vi "AlliGator Is SS2 Dataset HDF5 File.vi"(7 "File Path":path, 9 "Error In":errorcluster) -> (8 "Is SS2 Dataset?":bool, 10 "Error Out":errorcluster)   [LabVIEW 2021, in "AlliGator HDF5.lvlib"]
doc: "Checks wether a HDF5 file is a SS2 dataset file (early version)."
uses:
  AlliGator HDF5.lvlib
  <vilib>/addons/h5labview2/base/lib_path.vi
  <vilib>/addons/h5labview2/base/H5Equery.vi
  <vilib>/addons/h5labview2/base/hid_t.ctl
  <vilib>/addons/h5labview2/dataset/H5Dread.llb/H5Dread.xnode
  <vilib>/addons/h5labview2/file/H5F.lvlib
panel:
  # "see the AlliGator License on the block diagram (Ctrl+E or Window:Show Block Diagram)"
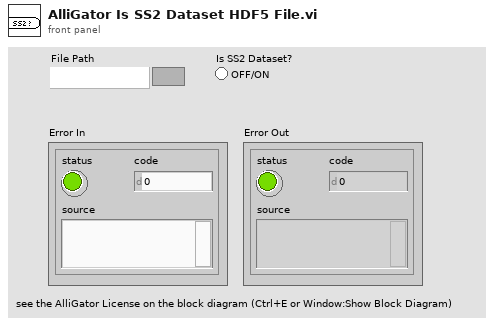
[diagram p1: front panel]
types:
  T1 = typedef "hid_t.ctl" = i64
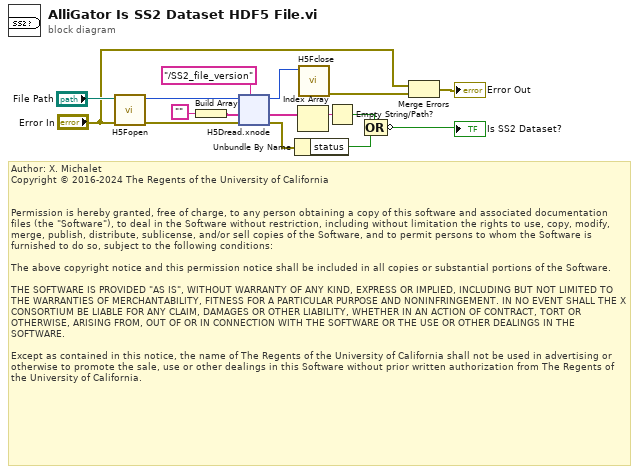
[diagram p0: block diagram]
diagram:
  # "Author: X. Michalet\nCopyright © 2016-2024 The Regents of the University of California\n \n\nPermission is hereby granted, free of charge, to any person obtaining a copy of this software and associated documentation files (the \"Software\"), to deal in the Software without restriction, including without limitation the rights to use, copy, modify, merge, publish, distribute, sublicense, and/or sell copies of the Software, and to permit persons to whom the Software is furnished to do so, subject to the following conditions:\n\nThe above copyright notice and this permission notice shall be included in all copies or substantial portions of the Software.\n\nTHE SOFTWARE IS PROVIDED \"AS IS\", WITHOUT WARRANTY OF ANY KIND, EXPRESS OR IMPLIED, INCLUDING BUT NOT LIMITED TO THE WARRANTIES OF MERCHANTABILITY, FITNESS FOR A PARTICULAR PURPOSE AND NONINFRINGEMENT. IN NO EVENT SHALL THE X CONSORTIUM BE LIABLE FOR ANY CLAIM, DAMAGES OR OTHER LIABILITY, WHETHER IN AN ACTION OF CONTRACT, TORT OR OTHERWISE, ARISING FROM, OUT OF OR IN CONNECTION WITH THE SOFTWARE OR THE USE OR OTHER DEALINGS IN THE SOFTWARE.\n\nExcept as contained in this notice, the name of The Regents of the University of California shall not be used in advertising or otherwise to promote the sale, use or other dealings in this Software without prior written authorization from The Regents of the University of California."
  n1 = call <vilib>:"H5Fopen.vi"("error in (no error)"="Error In", "path"="File Path") -> ("error out"=w12:errorcluster, "ref out"=w13:T1)  [unwired: 8 in]
  n2 = Build Array("") -> (w14:string[])
  n3 = xnode "H5Dread.xnode"("dataset name (this)"="/SS2_file_version", "error in (no error)"=w12, "default"=w14, "ref in"=w13) -> ("error out"=w9:errorcluster, "data"=w10:string[], "ref out"=w4:T1)  [unwired: 2 in, 1 out]
  n4 = Unbundle By Name(w9) -> ("status"=w7:bool)
  n5 = Index Array(array=w10) -> (element=w5:string)  [unwired: 1 in]
  n6 = call <vilib>:"H5Fclose.vi"("ref"=w4) -> ("error out"=w3:errorcluster)  [unwired: 10 in]
  n7 = Empty String/Path?(string/path=w5) -> (empty?=w8:bool)
  n8 = Compound Arithmetic op=OR(w8, w7) -> (invert →"Is SS2 Dataset?":bool)
  n9 = Merge Errors("Error In", w3) -> (→"Error Out":errorcluster)
